vi "TestCreateGreyscaleImage.vi"(8 "error in (no error)":errorcluster, 11 "Test Case In":refnum<class "Image.lvclass">) -> (0 "error out":errorcluster, 3 "Test Case Out":refnum<class "Image.lvclass">)   [LabVIEW 2020, in "g_ar_toolkit.test.lvlib" / "Image.lvclass"]
uses:
  Image.lvclass
  Image.lvclass/Image.ctl
  4993e8ee-a06a-463a-9684-69129f64d5ce.vi
  g_ar_toolkit.lvlib
  g_ar_toolkit/Image Size Cluster.ctl
  g_ar_toolkit/Create_Empty_Image_Greyscale.vi
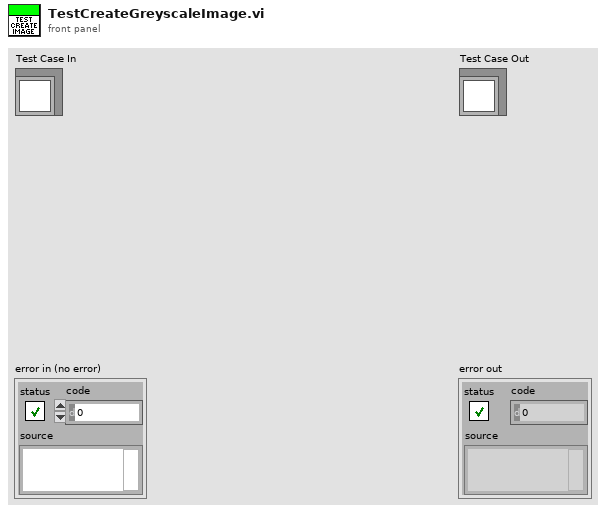
[diagram p1: front panel]
types:
  T1 = typedef "g_ar_toolkit.lvlib/Image Size Cluster.ctl" = cluster{"Width":u16, "Height":u16}
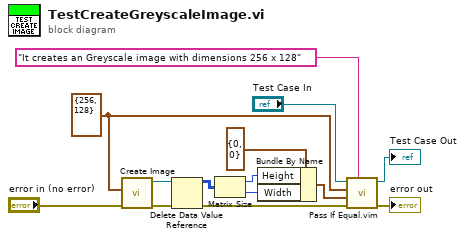
[diagram p0: block diagram]
diagram:
  w2 = T1 {"Width"=256, "Height"=128} ("Preallocated Image Size (Default - 0,0)")
  n1 = call-poly "Create Image.vi"("error in (no error)"="error in (no error)", "Preallocated Image Size (Default 0,0)"=w2) -> ("error out"=w9:errorcluster, "New Greyscale Image"=w10:refnum<data-value>)  [unwired: 8 in]
  n2 = Delete Data Value Reference(data value reference=w10, error in=w9) -> (data value=w7:u8[][], error out=w8:errorcluster)
  n3 = Matrix Size(0:w7) -> (1:w6:i32, 2:w5:i32)
  n4 = Bundle By Name(cluster=T1 {"Width"=0, "Height"=0} ("Preallocated Image Size (Default - 0,0)"), "Height"=w6, "Width"=w5) -> (w1:T1)
  n5 = call "Pass If Equal.vim"("Description"="It creates an Greyscale image with dimensions 256 x 128", "error in (no error)"=w8, "Actual"=w1, "Expected"=w2, "LUnit Test Case In"="Test Case In") -> ("error out"=→"error out":errorcluster, "LUnit Test Case Out"=→"Test Case Out":refnum<class "Image.lvclass">)  [unwired: 5 in]
